vi "test_libssh2_sftp_rmdir_ex.vi"() -> ()   [LabVIEW 2013, in "libssh2_integration_tests.lvlib"]
uses:
  libssh2_integration_tests.lvlib
  <vilib>/addons/_JKI Toolkits/Caraya/classes/Test/Test.lvclass
  support/support.lvlib
  <vilib>/addons/_JKI Toolkits/Caraya/classes/Assert/Assert.lvclass
  libssh2/libssh2.lvlib
panel:
  out "error out":errorcluster
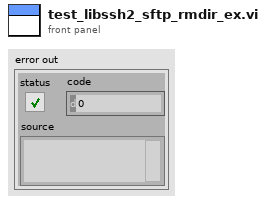
[diagram p1: front panel]
types:
  T1 = typedef "libssh2.lvlib/Session Refnum.ctl" = refnum<k1>
  T2 = typedef "libssh2.lvlib/SFTP Refnum.ctl" = refnum<k1>
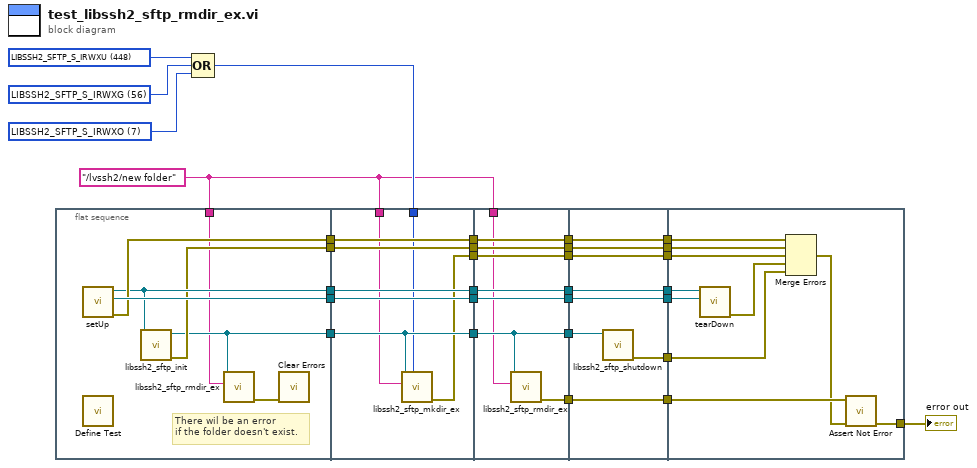
[diagram p0: block diagram]
diagram:
  w1 = "/lvssh2/new folder" ("filename")
  w23 = 7 items=["LIBSSH2_SFTP_S_IRWXU"=448, "LIBSSH2_SFTP_S_IRUSR"=256, "LIBSSH2_SFTP_S_IWUSR"=128, "LIBSSH2_SFTP_S_IXUSR"=64, "LIBSSH2_SFTP_S_IRWXG"=56, "LIBSSH2_SFTP_S_IRGRP"=32, "LIBSSH2_SFTP_S_IWGRP"=16, "LIBSSH2_SFTP_S_IXGRP"=8, "LIBSSH2_SFTP_S_IRWXO"=7, "LIBSSH2_SFTP_S_IROTH"=4, "LIBSSH2_SFTP_S_IWOTH"=2, "LIBSSH2_SFTP_S_IXOTH"=1] ("mode")
  w24 = 56 items=["LIBSSH2_SFTP_S_IRWXU"=448, "LIBSSH2_SFTP_S_IRUSR"=256, "LIBSSH2_SFTP_S_IWUSR"=128, "LIBSSH2_SFTP_S_IXUSR"=64, "LIBSSH2_SFTP_S_IRWXG"=56, "LIBSSH2_SFTP_S_IRGRP"=32, "LIBSSH2_SFTP_S_IWGRP"=16, "LIBSSH2_SFTP_S_IXGRP"=8, "LIBSSH2_SFTP_S_IRWXO"=7, "LIBSSH2_SFTP_S_IROTH"=4, "LIBSSH2_SFTP_S_IWOTH"=2, "LIBSSH2_SFTP_S_IXOTH"=1] ("mode")
  w25 = 448 items=["LIBSSH2_SFTP_S_IRWXU"=448, "LIBSSH2_SFTP_S_IRUSR"=256, "LIBSSH2_SFTP_S_IWUSR"=128, "LIBSSH2_SFTP_S_IXUSR"=64, "LIBSSH2_SFTP_S_IRWXG"=56, "LIBSSH2_SFTP_S_IRGRP"=32, "LIBSSH2_SFTP_S_IWGRP"=16, "LIBSSH2_SFTP_S_IXGRP"=8, "LIBSSH2_SFTP_S_IRWXO"=7, "LIBSSH2_SFTP_S_IROTH"=4, "LIBSSH2_SFTP_S_IWOTH"=2, "LIBSSH2_SFTP_S_IXOTH"=1] ("mode")
  n1 = flat-sequence {
    tunnel: [w36] -> w31
    tunnel: [w38] -> w30
    tunnel: [w37] -> w29
    tunnel: [w35] -> w27
    tunnel: [w34] -> w26
    tunnel: w1 -> [w33]
    tunnel: w31 -> [w46]
    tunnel: w30 -> [w45]
    tunnel: [w46] -> w15
    tunnel: [w45] -> w13
    tunnel: [w42] -> w11
    tunnel: [w44] -> w8
    tunnel: w29 -> [w44]
    tunnel: w27 -> [w43]
    tunnel: [w43] -> w6
    tunnel: w26 -> [w42]
    tunnel: w22 -> [w41]
    tunnel: w1 -> [w40]
    tunnel: [w39] -> w4
    tunnel: w15 -> [w54]
    tunnel: [w54] -> w14
    tunnel: w13 -> [w53]
    tunnel: [w53] -> w12
    tunnel: w11 -> [w48]
    tunnel: [w48] -> w10
    tunnel: [w49] -> w9
    tunnel: w8 -> [w52]
    tunnel: [w52] -> w7
    tunnel: w6 -> [w51]
    tunnel: [w51] -> w5
    tunnel: w4 -> [w50]
    tunnel: [w50] -> w3
    tunnel: w1 -> [w47]
    tunnel: w14 -> [w62]
    tunnel: [w62] -> w21
    tunnel: w12 -> [w61]
    tunnel: [w61] -> w20
    tunnel: w10 -> [w57]
    tunnel: w9 -> [w60]
    tunnel: [w60] -> w19
    tunnel: w7 -> [w59]
    tunnel: [w59] -> w18
    tunnel: w5 -> [w58]
    tunnel: [w58] -> w17
    tunnel: [w56] -> w16
    tunnel: w3 -> [w55]
    tunnel: [w55] -> w2
    tunnel: w21 -> [w72]
    tunnel: w20 -> [w71]
    tunnel: w19 -> [w70]
    tunnel: w18 -> [w69]
    tunnel: [w66] -> w28
    tunnel: w17 -> [w65]
    tunnel: w16 -> [w64]
    tunnel: w2 -> [w63]
    frame #0 {
      # "There wil be an error\nif the folder doesn't exist."
      n2 = call "setUp.vi"() -> ("error out"=w37:errorcluster, "connection ID"=w38:refnum<k5>, "session"=w36:T1)  [unwired: 9 in]
      n3 = call <vilib>:"Define Test.vi"() -> ()  [unwired: 10 in, 2 out]
      n4 = call "libssh2_sftp_init.vi"("session"=w36) -> ("error out"=w35:errorcluster, "sftp"=w34:T2)  [unwired: 9 in]
      n5 = call "libssh2_sftp_rmdir_ex.vi"("path"=w33, "sftp"=w34) -> ("error out"=w32:errorcluster)  [unwired: 9 in]
      n6 = call <vilib>:"Clear Errors.vi"("error in (no error)"=w32) -> ()  [unwired: 6 in, 1 out]
    }
    frame #1 {
      n7 = call "libssh2_sftp_mkdir_ex.vi"("mode"=w41, "path"=w40, "sftp"=w42) -> ("error out"=w39:errorcluster)  [unwired: 8 in]
    }
    frame #2 {
      n8 = call "libssh2_sftp_rmdir_ex.vi"("path"=w47, "sftp"=w48) -> ("error out"=w49:errorcluster)  [unwired: 9 in]
    }
    frame #3 {
      n9 = call "libssh2_sftp_shutdown.vi"("sftp"=w57) -> ("error out"=w56:errorcluster)  [unwired: 10 in]
    }
    frame #4 {
      n10 = call "tearDown.vi"("connection ID"=w71, "session"=w72) -> ("error out"=w68:errorcluster)  [unwired: 9 in]
      n11 = Merge Errors(w69, w65, w63, w68, w64) -> (w67:errorcluster)
      n12 = call <vilib>:"Assert Not Error.vi"("error in (no error)"=w67, "Not Error?"=w70) -> ("error out"=w66:errorcluster)  [unwired: 8 in, 1 out]
    }
  }
  n13 = Compound Arithmetic op=OR(w25, w24, w23) -> (w22:i32)
  "error out" <- w28
